vi "Save File Create Filename.vi"(7 "LV Program":T1=enum."DOE Stand", 8 "Error In":errorcluster, 11 "Initialize.Washer In":T2={"Appliance Details"={"FileVersionInfo"={"FileVersion"="", "ProductName"="", "InternalName"="", "CompanyName"="", "LegalCopyright"="", "FileDescription"=""}, "Dishwasher Info"={"Open Cup Weight (gm):"=0.0, "Auto Cup Weight (gm):"=0.0, "Detergent-Dish:"="", "Inlet Temperature-Dish:"="", "Cycle Mode-Dish:"="", "Unit Control-Dish:"="", "Manufacturer-Dish:"=""}, "Washer Info"={"Hot Water Temperature (Fahrenheit):"="", "Cold Water Temperature (Fahrenheit):"="", "Capacity (cu.ft):"=0.0, "Initial Cloth Weight:"=0.0, "Cloth Lot:"=0, "Model Family:"="", "Program Name:"="", "Cycle Selection:"="", "Wash Temperature:"="", "Rinse Temperature:"="", "Load Size:"=""}, "File Name Output Array"=[], "Calibration Output Array"=[], "Appliance Common"={"Engineer:"="", "Model Number:"="", "Serial Number:"="", "Comments:"="", "Station ID:"="", "Technician:"="", "TR Number:"="", "Lab ID:"="", "Voltage:"="", "Water Pressure (PSI):"="", "Test Date:"="", "Computer Name:"="", "IP Address:"="", "Ambient RH:"="", "Frequency:"="", "Build:"="", "Filename:"="", "Test Type:"="", "Load Run #:"=0, "Ambient Temperature (F):"="", "File Path:"=path "", "Cycles Per Year"=0}, "Water Heater"={"Heating Mode:"=""}, "Dryer"={"Heat Setting:"="", "Washer Water Temperature (60 ± 5°F):"=0, "Water Hardness (PPM):"=0, "Dryness Setting:"="", "Dryer Type:"="", "Exhaust:"="", "Drying Cycle:"="", "Load Type:"="", "Nominal Load Weight"="", "Dryer Initial IMC Data"={"Measured IMC (lbs)"=0.0, "Actual Initial RMC (%)"=0.0, "RMC (Desired %)"=0.0, "Bone Dry Wt(lbs)"=0.0, "Tolerance(%)"=0.0, "Actual Final RMC (%)"=7.0, "CEF (lbf/kWh)"=0.0, "Minimum Weight (lbf)"=0.0, "Average Weight (lbf)"=0.0, "Maximum Weight (lbf)"=0.0, "Measured IMC In Range?"=FALSE, "Moisture Reduction Factor"=55.5, "Field Use Factor"=1.04, "Empty Dryer Cold Weigth"=0.0, "Energy Standard"=enum."D2-Automatic Dryer", "Weight Cloth (lbs)"=0.0, "Relative Moisture Content (%)"=0.0, "Relative Moisture Content - Avg (%)"=0.0}}}, "Display Data (RLT)"={"Status Color"=0, "Serial Number Display"="", "Cycle Count Display"=0, "Station Label Display"="", "Current Run Start Time Display"=0.0, "Board ID Display"="", "RPM Display"=0, "Current Display"=0.0, "Current Path Display"=path "", "Saving Display"=FALSE, "Unit Type Display"=enum."", "Total Time On Display"=0.0, "UI Button"=FALSE}} {"Display Data (RLT)"."Current Display" format="%.2f"; "Display Data (RLT)"."Cycle Count Display" format="%04d"; "Appliance Details"."Dryer"."Dryer Initial IMC Data"."Maximum Weight (lbf)" format="%03_6g"; "Appliance Details"."Dryer"."Dryer Initial IMC Data"."Average Weight (lbf)" format="%03_6g"; "Appliance Details"."Dryer"."Dryer Initial IMC Data"."Minimum Weight (lbf)" format="%03_6g"; "Appliance Details"."Dryer"."Dryer Initial IMC Data"."CEF (lbf/kWh)" format="%03_6g"; "Appliance Details"."Dryer"."Dryer Initial IMC Data"."Actual Final RMC (%)" format="%03_6g"; "Appliance Details"."Dryer"."Dryer Initial IMC Data"."Tolerance(%)" format="%0#_6g"; "Appliance Details"."Dryer"."Dryer Initial IMC Data"."Bone Dry Wt(lbs)" format="%03_6g"; "Appliance Details"."Dryer"."Dryer Initial IMC Data"."RMC (Desired %)" format="%0#_6g"; "Appliance Details"."Dryer"."Dryer Initial IMC Data"."Actual Initial RMC (%)" format="%03_6g"; "Appliance Details"."Dryer"."Dryer Initial IMC Data"."Measured IMC (lbs)" format="%0#_6g"}) -> (0 "Error Out":errorcluster, 2 "Filename":string, 3 "Initialize.Washer Out":T2={"Appliance Details"={"FileVersionInfo"={"FileVersion"="", "ProductName"="", "InternalName"="", "CompanyName"="", "LegalCopyright"="", "FileDescription"=""}, "Dishwasher Info"={"Open Cup Weight (gm):"=0.0, "Auto Cup Weight (gm):"=0.0, "Detergent-Dish:"="", "Inlet Temperature-Dish:"="", "Cycle Mode-Dish:"="", "Unit Control-Dish:"="", "Manufacturer-Dish:"=""}, "Washer Info"={"Hot Water Temperature (Fahrenheit):"="", "Cold Water Temperature (Fahrenheit):"="", "Capacity (cu.ft):"=0.0, "Initial Cloth Weight:"=0.0, "Cloth Lot:"=0, "Model Family:"="", "Program Name:"="", "Cycle Selection:"="", "Wash Temperature:"="", "Rinse Temperature:"="", "Load Size:"=""}, "File Name Output Array"=[], "Calibration Output Array"=[], "Appliance Common"={"Engineer:"="", "Model Number:"="", "Serial Number:"="", "Comments:"="", "Station ID:"="", "Technician:"="", "TR Number:"="", "Lab ID:"="", "Voltage:"="", "Water Pressure (PSI):"="", "Test Date:"="", "Computer Name:"="", "IP Address:"="", "Ambient RH:"="", "Frequency:"="", "Build:"="", "Filename:"="", "Test Type:"="", "Load Run #:"=0, "Ambient Temperature (F):"="", "File Path:"=path "", "Cycles Per Year"=0}, "Water Heater"={"Heating Mode:"=""}, "Dryer"={"Heat Setting:"="", "Washer Water Temperature (60 ± 5°F):"=0, "Water Hardness (PPM):"=0, "Dryness Setting:"="", "Dryer Type:"="", "Exhaust:"="", "Drying Cycle:"="", "Load Type:"="", "Nominal Load Weight"="", "Dryer Initial IMC Data"={"Measured IMC (lbs)"=0.0, "Actual Initial RMC (%)"=0.0, "RMC (Desired %)"=0.0, "Bone Dry Wt(lbs)"=0.0, "Tolerance(%)"=0.0, "Actual Final RMC (%)"=7.0, "CEF (lbf/kWh)"=0.0, "Minimum Weight (lbf)"=0.0, "Average Weight (lbf)"=0.0, "Maximum Weight (lbf)"=0.0, "Measured IMC In Range?"=FALSE, "Moisture Reduction Factor"=55.5, "Field Use Factor"=1.04, "Empty Dryer Cold Weigth"=0.0, "Energy Standard"=enum."D2-Automatic Dryer", "Weight Cloth (lbs)"=0.0, "Relative Moisture Content (%)"=0.0, "Relative Moisture Content - Avg (%)"=0.0}}}, "Display Data (RLT)"={"Status Color"=0, "Serial Number Display"="", "Cycle Count Display"=0, "Station Label Display"="", "Current Run Start Time Display"=0.0, "Board ID Display"="", "RPM Display"=0, "Current Display"=0.0, "Current Path Display"=path "", "Saving Display"=FALSE, "Unit Type Display"=enum."", "Total Time On Display"=0.0, "UI Button"=FALSE}} {"Display Data (RLT)"."Current Display" format="%.2f"; "Display Data (RLT)"."Cycle Count Display" format="%04d"; "Appliance Details"."Dryer"."Dryer Initial IMC Data"."Maximum Weight (lbf)" format="%03_6g"; "Appliance Details"."Dryer"."Dryer Initial IMC Data"."Average Weight (lbf)" format="%03_6g"; "Appliance Details"."Dryer"."Dryer Initial IMC Data"."Minimum Weight (lbf)" format="%03_6g"; "Appliance Details"."Dryer"."Dryer Initial IMC Data"."CEF (lbf/kWh)" format="%03_6g"; "Appliance Details"."Dryer"."Dryer Initial IMC Data"."Actual Final RMC (%)" format="%03_6g"; "Appliance Details"."Dryer"."Dryer Initial IMC Data"."Tolerance(%)" format="%0#_6g"; "Appliance Details"."Dryer"."Dryer Initial IMC Data"."Bone Dry Wt(lbs)" format="%03_6g"; "Appliance Details"."Dryer"."Dryer Initial IMC Data"."RMC (Desired %)" format="%0#_6g"; "Appliance Details"."Dryer"."Dryer Initial IMC Data"."Actual Initial RMC (%)" format="%03_6g"; "Appliance Details"."Dryer"."Dryer Initial IMC Data"."Measured IMC (lbs)" format="%0#_6g"})   [LabVIEW 2023, in "Save File.lvlib"]
uses:
  Save File.lvlib
  Public/Type Definitions/Save File Washer.ctl
  File Setup (Public)/Type Definition/Save File DISH Dishwasher Details.ctl
  <vilib>/Platform/fileVersionInfo.llb/FileVersionInformation.ctl
  Washer DOE/Type Definitions/DOE Appliance Common.ctl
  Custom Pallet Controls/Custom Pallet String.ctl
  File Setup (Public)/Type Definition/DPT IMC Data.ctl
  Washer DOE/Type Definitions/DOE Dryer Standard.ctl
  Public/Type Definitions/Save File Appliance Display.ctl
  Public/Type Definitions/Save File Unit Type.ctl
  File Setup (Public)/Type Definition/Save File DOE LabView Program.ctl
  File Setup.lvlib
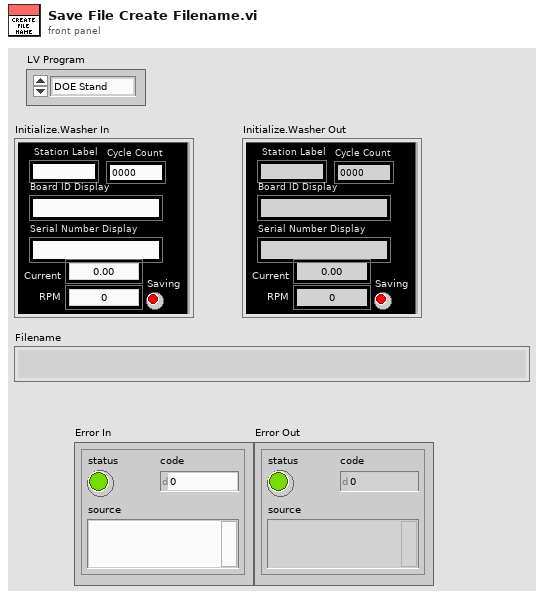
[diagram p1: front panel]
types:
  T1 = typedef "File Setup.lvlib/Save File DOE LabView Program.ctl" = enum16{"No Name Found", "DOE Stand", "Dishwasher Kitchen", "Portable Stand", "HEWH", "Dryer", "Dryer WILT", "HCC", "PRAT", "HEWH RLT", "Refrigeration", "Gas Water Heater"}
  T2 = typedef "Save File.lvlib/Save File Washer.ctl" = cluster{"Appliance Details":T3, "Display Data (RLT)":T9}
  T3 = typedef "File Setup.lvlib/Save File DISH Dishwasher Details.ctl" = cluster{"FileVersionInfo":T4, "Dishwasher Info":cluster{"Open Cup Weight (gm):":dbl, "Auto Cup Weight (gm):":dbl, "Detergent-Dish:":string, "Inlet Temperature-Dish:":string, "Cycle Mode-Dish:":string, "Unit Control-Dish:":string, "Manufacturer-Dish:":string}, "Washer Info":cluster{"Hot Water Temperature (Fahrenheit):":string, "Cold Water Temperature (Fahrenheit):":string, "Capacity (cu.ft):":dbl, "Initial Cloth Weight:":dbl, "Cloth Lot:":i32, "Model Family:":string, "Program Name:":string, "Cycle Selection:":string, "Wash Temperature:":string, "Rinse Temperature:":string, "Load Size:":string}, "File Name Output Array":string[][], "Calibration Output Array":string[][], "Appliance Common":T5, "Water Heater":cluster{"Heating Mode:":string}, "Dryer":cluster{"Heat Setting:":T6, "Washer Water Temperature (60 ± 5°F):":u16, "Water Hardness (PPM):":u16, "Dryness Setting:":T6, "Dryer Type:":string, "Exhaust:":string, "Drying Cycle:":string, "Load Type:":string, "Nominal Load Weight":string, "Dryer Initial IMC Data":T7}}
  T4 = typedef "FileVersionInformation.ctl" = cluster{"FileVersion":string, "ProductName":string, "InternalName":string, "CompanyName":string, "LegalCopyright":string, "FileDescription":string}
  T5 = typedef "DOE Appliance Common.ctl" = cluster{"Engineer:":string, "Model Number:":string, "Serial Number:":string, "Comments:":string, "Station ID:":string, "Technician:":string, "TR Number:":string, "Lab ID:":string, "Voltage:":string, "Water Pressure (PSI):":string, "Test Date:":string, "Computer Name:":string, "IP Address:":string, "Ambient RH:":string, "Frequency:":string, "Build:":string, "Filename:":string, "Test Type:":string, "Load Run #:":i32, "Ambient Temperature (F):":string, "File Path:":path, "Cycles Per Year":u32}
  T6 = typedef "Custom Pallet String.ctl" = string
  T7 = typedef "DPT IMC Data.ctl" = cluster{"Measured IMC (lbs)":dbl, "Actual Initial RMC (%)":dbl, "RMC (Desired %)":dbl, "Bone Dry Wt(lbs)":dbl, "Tolerance(%)":dbl, "Actual Final RMC (%)":dbl, "CEF (lbf/kWh)":dbl, "Minimum Weight (lbf)":dbl, "Average Weight (lbf)":dbl, "Maximum Weight (lbf)":dbl, "Measured IMC In Range?":bool, "Moisture Reduction Factor":dbl, "Field Use Factor":dbl, "Empty Dryer Cold Weigth":dbl, "Energy Standard":T8, "Weight Cloth (lbs)":dbl, "Relative Moisture Content (%)":dbl, "Relative Moisture Content - Avg (%)":dbl}
  T8 = typedef "DOE Dryer Standard.ctl" = enum16{"D2-Automatic Dryer", "D2-Timer Dryer", "D1-Automatic Dryer", "D1-Timer Dryer", "Other"}
  T9 = typedef "Save File Appliance Display.ctl" = cluster{"Status Color":u32, "Serial Number Display":string, "Cycle Count Display":i32, "Station Label Display":string, "Current Run Start Time Display":dbl, "Board ID Display":string, "RPM Display":u32, "Current Display":dbl, "Current Path Display":path, "Saving Display":bool, "Unit Type Display":T10, "Total Time On Display":dbl, "UI Button":bool}
  T10 = typedef "Save File.lvlib/Save File Unit Type.ctl" = enum32{"", "Viper", "Hawk", "2015"}
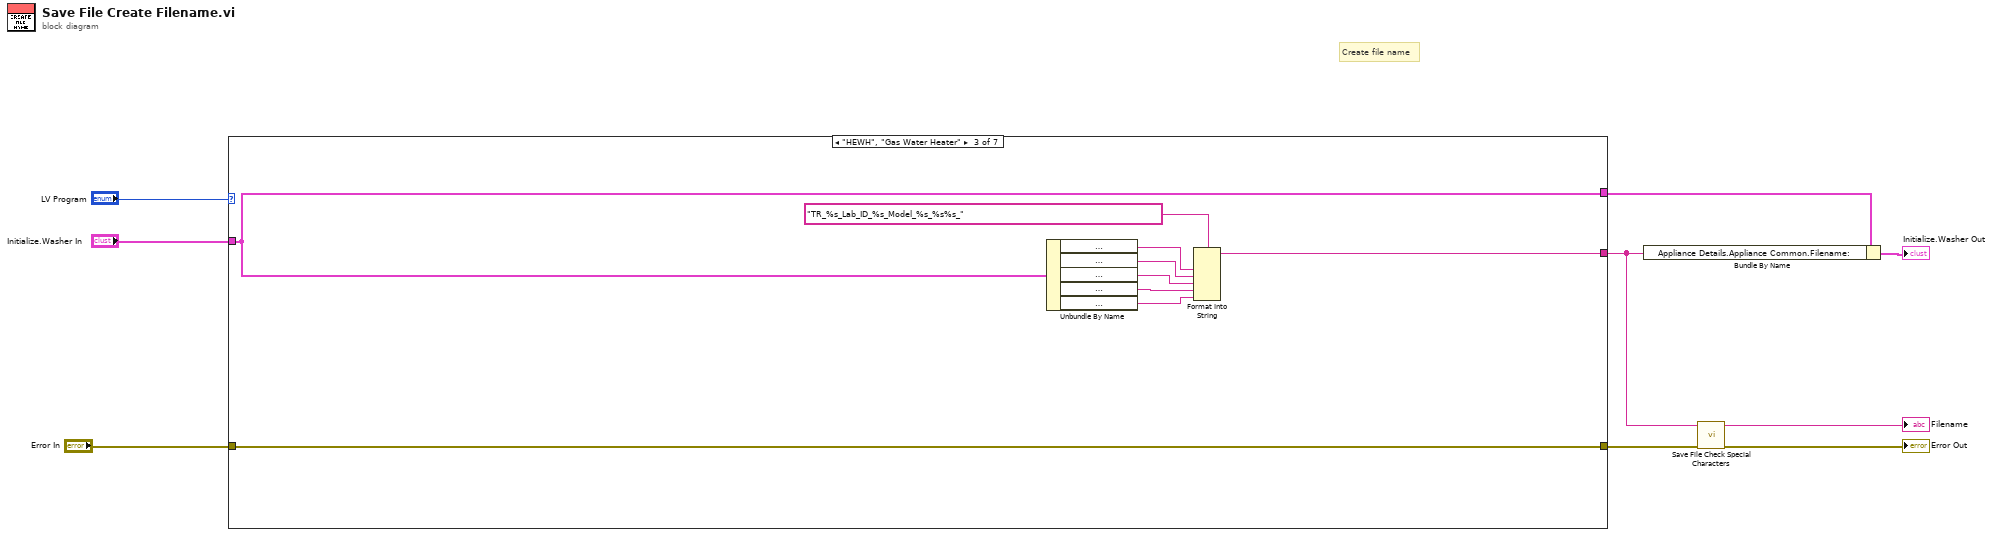
[diagram p0: block diagram]
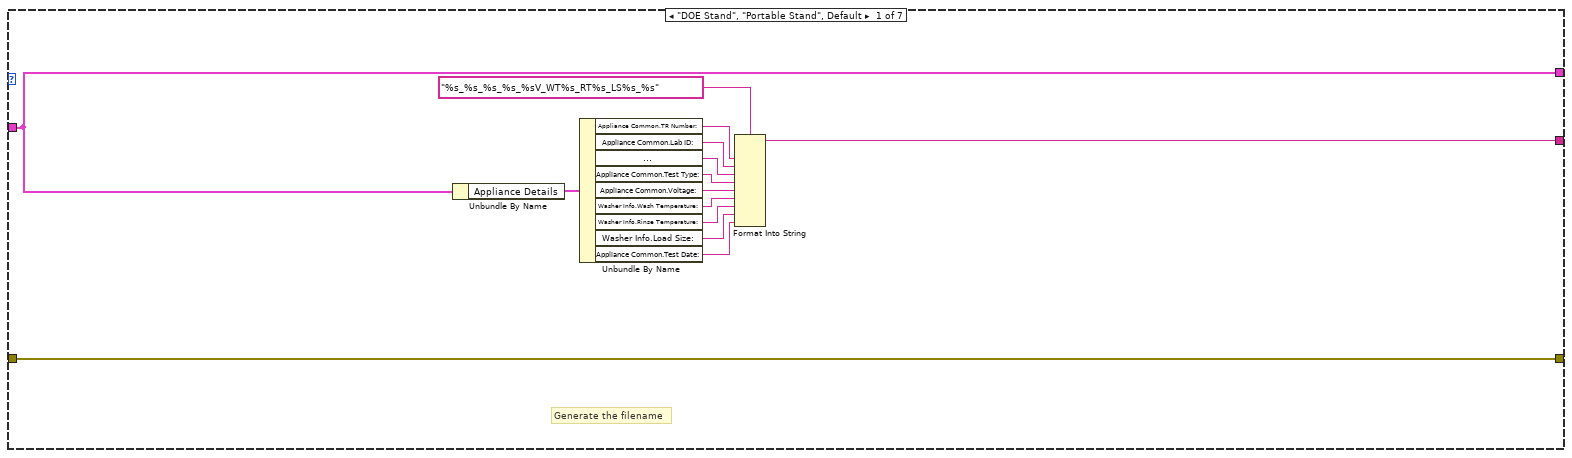
[diagram p2: hidden frame]
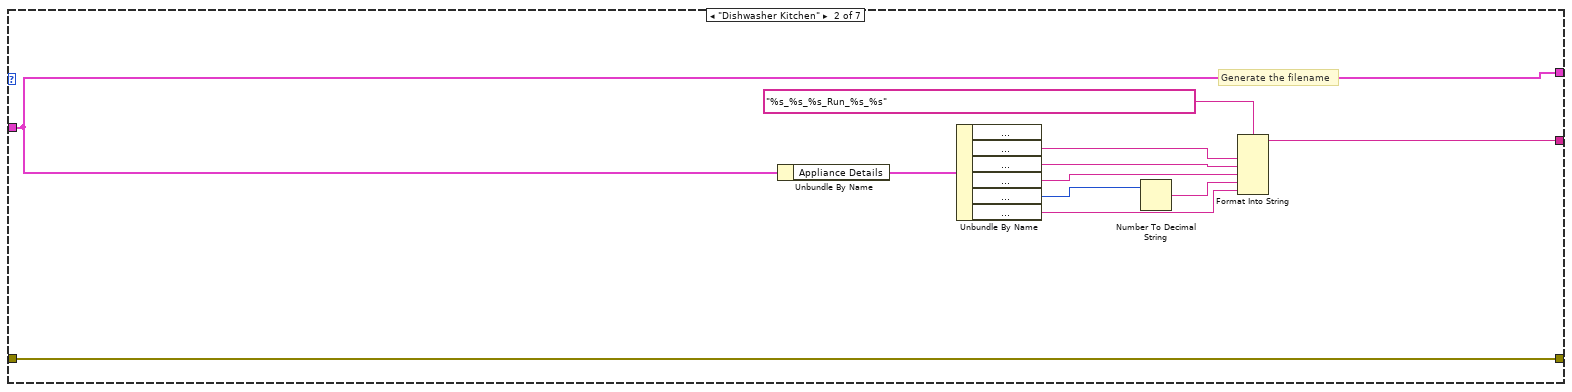
[diagram p3: hidden frame]
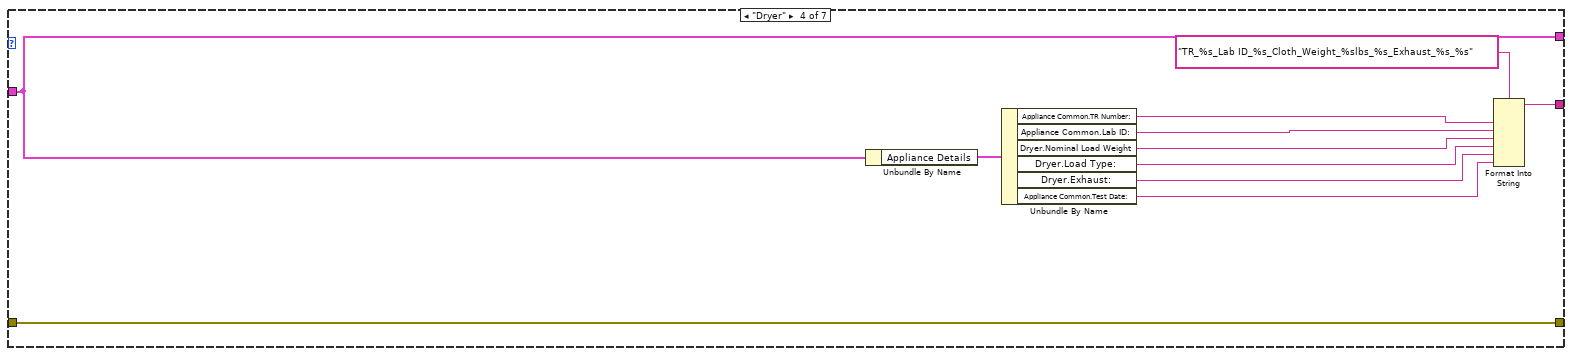
[diagram p4: hidden frame]
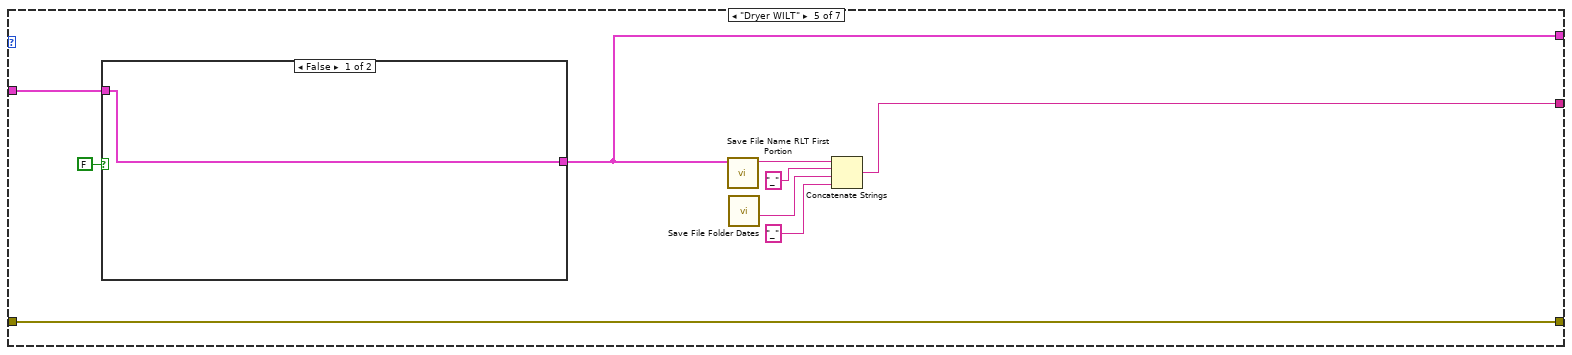
[diagram p5: hidden frame]
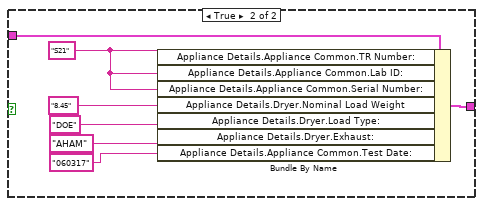
[diagram p6: hidden frame]
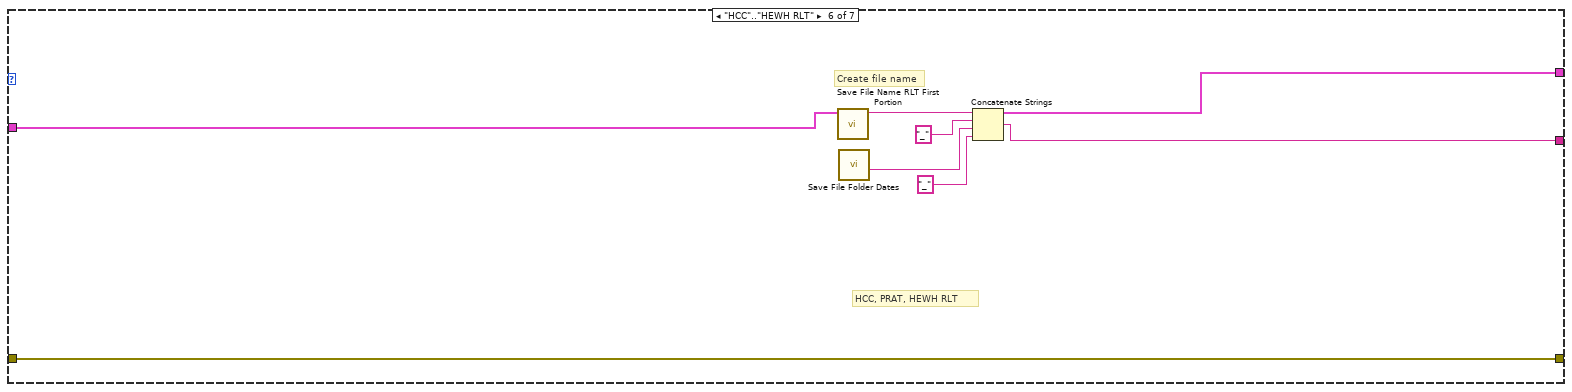
[diagram p7: hidden frame]
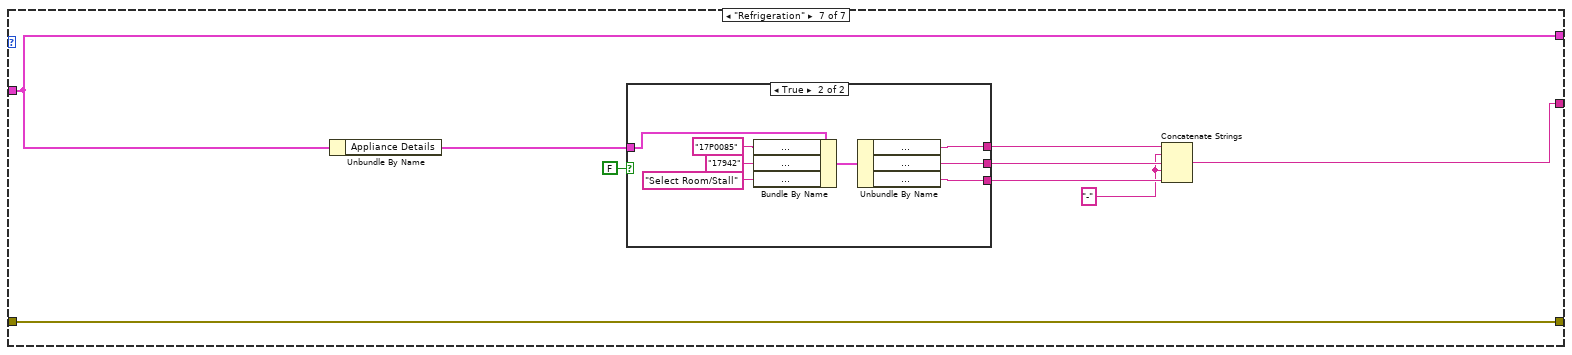
[diagram p8: hidden frame]
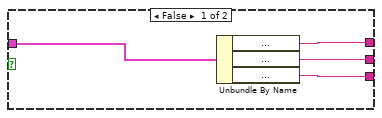
[diagram p9: hidden frame]
diagram:
  # "Create file name"
  n1 = case shown="\"HEWH\", \"Gas Water Heater\"" "LV Program" {
    tunnel: [w23 w31 w42 w49 w60 w74 w85] -> w4
    tunnel: [w10 w24 w35 w44 w57 w75 w84] -> w6
    tunnel: "Error In" -> [w12 w26 w41 w48 w63 w78 w83]
    tunnel: [w12 w26 w41 w48 w63 w78 w83] -> w2
    tunnel: "Initialize.Washer In" -> [w10 w24 w35 w44 w62 w75 w84]
    frame "DOE Stand", "Portable Stand", Default {
      # "Generate the filename"
      n2 = Unbundle By Name(w10) -> ("Appliance Details"=w11:T3)
      n3 = Unbundle By Name(w11) -> ("Appliance Common.TR Number:"=w22:string, "Appliance Common.Lab ID:"=w21:string, "Appliance Common.Model Number:"=w19:string, "Appliance Common.Test Type:"=w13:string, "Appliance Common.Voltage:"=w20:string, "Washer Info.Wash Temperature:"=w17:string, "Washer Info.Rinse Temperature:"=w16:string, "Washer Info.Load Size:"=w15:string, "Appliance Common.Test Date:"=w14:string)
      n4 = Format Into String(format string="%s_%s_%s_%s_%sV_WT%s_RT%s_LS%s_%s", w22, w21, w19, w13, w20, w17, w16, w15, w14) -> (resulting string=w23:string)  [unwired: 2 in, 1 out]
    }
    frame "Dishwasher Kitchen" {
      # "Generate the filename"
      n5 = Unbundle By Name(w24) -> ("Appliance Details"=w25:T3)
      n6 = Unbundle By Name(w25) -> ("Appliance Common.Lab ID:"=w32:string, "Appliance Common.Test Type:"=w33:string, "Appliance Common.Comments:"=w34:string, "Appliance Common.Load Run #:"=w28:i32, "Appliance Common.Test Date:"=w29:string)  [unwired: 1 out]
      n7 = Number To Decimal String(number=w28) -> (decimal integer string=w27:string)  [unwired: 1 in]
      n8 = Format Into String(format string="%s_%s_%s_Run_%s_%s", w32, w33, w34, w27, w29) -> (resulting string=w31:string)  [unwired: 2 in, 1 out]
    }
    frame "HEWH", "Gas Water Heater" {
      n9 = Unbundle By Name(w35) -> ("Appliance Details.Appliance Common.TR Number:"=w40:string, "Appliance Details.Appliance Common.Lab ID:"=w39:string, "Appliance Details.Appliance Common.Model Number:"=w38:string, "Appliance Details.Appliance Common.Test Date:"=w37:string, "Appliance Details.Appliance Common.Test Type:"=w36:string)
      n10 = Format Into String(format string="TR_%s_Lab_ID_%s_Model_%s_%s%s_", w40, w39, w38, w37, w36) -> (resulting string=w42:string)  [unwired: 2 in, 1 out]
    }
    frame "Dryer" {
      n11 = Unbundle By Name(w44) -> ("Appliance Details"=w47:T3)
      n12 = Unbundle By Name(w47) -> ("Appliance Common.TR Number:"=w46:string, "Appliance Common.Lab ID:"=w45:string, "Dryer.Nominal Load Weight"=w50:string, "Dryer.Load Type:"=w51:string, "Dryer.Exhaust:"=w52:string, "Appliance Common.Test Date:"=w53:string)
      n13 = Format Into String(format string="TR_%s_Lab ID_%s_Cloth_Weight_%slbs_%s_Exhaust_%s_%s", w46, w45, w50, w51, w52, w53) -> (resulting string=w49:string)  [unwired: 2 in, 1 out]
    }
    frame "Dryer WILT" {
      n14 = case shown="False" FALSE {
        tunnel: w62 -> [w64 w66]
        tunnel: [w64 w65] -> w57
        frame False {
        }
        frame True {
          w71 = "S21" ("Appliance Details.Appliance Common.TR Number:")
          n15 = Bundle By Name(cluster=w66, "Appliance Details.Appliance Common.TR Number:"=w71, "Appliance Details.Appliance Common.Lab ID:"=w71, "Appliance Details.Appliance Common.Serial Number:"=w71, "Appliance Details.Dryer.Nominal Load Weight"="8.45", "Appliance Details.Dryer.Load Type:"="DOE", "Appliance Details.Dryer.Exhaust:"="AHAM", "Appliance Details.Appliance Common.Test Date:"="060317") -> (w65:T2)
        }
      }
      n16 = call "Save File Name RLT First Portion.vi"("Initialize.Washer In"=w57) -> ("Filename"=w61:string)  [unwired: 9 in, 1 out]
      n17 = call "Save File Folder Dates.vi"() -> ("Year/Month/Day"=w56:string)  [unwired: 8 in, 3 out]
      n18 = Concatenate Strings(w61, "_" ("string"), w56, "_" ("string")) -> (w60:string)
    }
    frame "HCC".."HEWH RLT" {
      # "HCC, PRAT, HEWH RLT"
      # "Create file name"
      n19 = call "Save File Name RLT First Portion.vi"("Initialize.Washer In"=w75) -> ("Filename"=w77:string)  [unwired: 9 in, 1 out]
      n20 = call "Save File Folder Dates.vi"() -> ("Year/Month/Day"=w72:string)  [unwired: 8 in, 3 out]
      n21 = Concatenate Strings(w77, "_" ("string"), w72, "_" ("string")) -> (w74:string)
    }
    frame "Refrigeration" {
      w79 = "-" ("string")
      n22 = Unbundle By Name(w84) -> ("Appliance Details"=w87:T3)
      n23 = case shown="True" FALSE {
        tunnel: w87 -> [w91 w99]
        tunnel: [w90 w96] -> w86
        tunnel: [w89 w95] -> w81
        tunnel: [w88 w94] -> w80
        frame False {
          n24 = Unbundle By Name(w91) -> ("Appliance Common.Lab ID:"=w90:string, "Appliance Common.TR Number:"=w89:string, "Appliance Common.Station ID:"=w88:string)
        }
        frame True {
          n25 = Bundle By Name(cluster=w99, "Appliance Common.Lab ID:"="17P0085" ("Appliance Common.TR Number:"), "Appliance Common.TR Number:"="17942", "Appliance Common.Station ID:"="Select Room/Stall" ("Appliance Common.TR Number:")) -> (w97:T3)
          n26 = Unbundle By Name(w97) -> ("Appliance Common.Lab ID:"=w96:string, "Appliance Common.TR Number:"=w95:string, "Appliance Common.Station ID:"=w94:string)
        }
      }
      n27 = Concatenate Strings(w86, w79, w81, w79, w80) -> (w85:string)
    }
  }
  n28 = Bundle By Name(cluster=w6, "Appliance Details.Appliance Common.Filename:"=w4) -> (→"Initialize.Washer Out":T2)
  n29 = call "Save File Check Special Characters.vi"("Error In"=w2, "Filename"=w4) -> ("Error Out"=→"Error Out":errorcluster, "Filename Output"=→"Filename":string)  [unwired: 8 in]
